vi "Publish Sample.vi"(8 "error in (no error)":errorcluster, 9 "Sample":refnum<class "Sample.lvclass">, 10 "Indice":i32[](array[numeric]), 11 "Storage Line in":refnum<class "Storage Line.lvclass">) -> (0 "error out":errorcluster, 3 "Storage Line out":refnum<class "Storage Line.lvclass">)   [LabVIEW 2015, in "cRIO-Carbondioxide.lvlib" / "CO2-Actor.lvlib" / "Storage Line.lvclass"]
uses:
  Storage Line.lvclass
  subs/Sample/Sample.lvclass
  Storage Line.lvclass/Storage Line.ctl
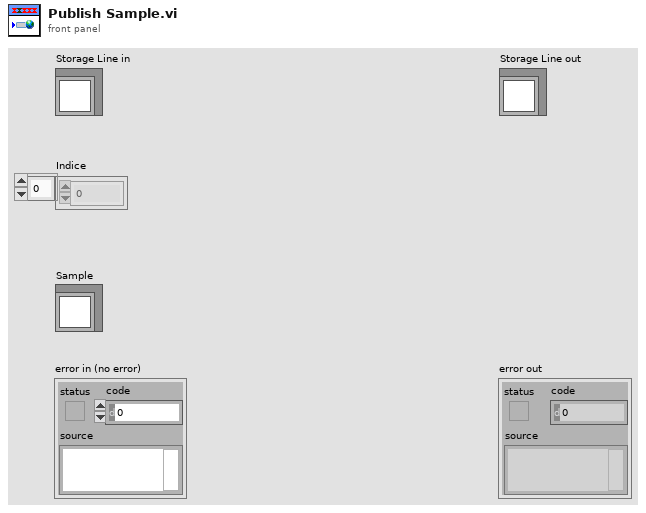
[diagram p1: front panel]
types:
  T1 = typedef "Sample Container.ctl" = cluster{"Sample In":refnum<k21>, "Sample Name":refnum<k21>, "Ti Cathode":refnum<k21>, "SampleQ":refnum<queue>}
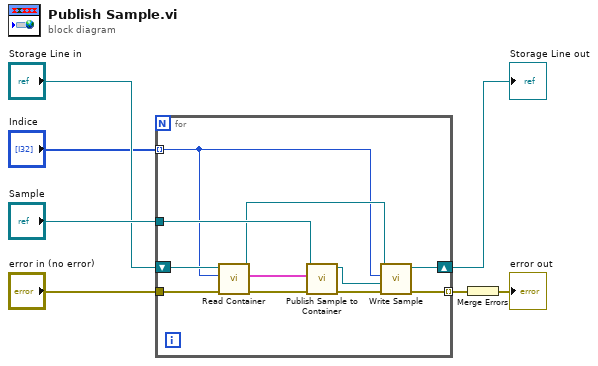
[diagram p0: block diagram]
diagram:
  n1 = for {
    tunnel: "Sample" -> [w18]
    shift-right: [w11] -> w4
    shift-left: "Storage Line in" -> [w12]
    tunnel: "Indice" -> [w9] mode=indexing
    tunnel: "error in (no error)" -> [w17]
    tunnel: [w14] -> w5 mode=indexing
    n2 = call "Read Container.vi"("error in (no error)"=w17, "index"=w9, "Storage Line in"=w12) -> ("error out"=w16:errorcluster, "Containers"=w8:T1[], "Storage Line out"=w10:refnum<class "Storage Line.lvclass">)  [unwired: 5 in, 1 out]
    n3 = call "Publish Sample to Container.vi"("error in (no error)"=w16, "Containers"=w8, "Sample in"=w18) -> ("error out"=w15:errorcluster, "Sample out"=w13:refnum<class "Sample.lvclass">)  [unwired: 7 in]
    n4 = call "Write Sample.vi"("error in (no error)"=w15, "Sample"=w13, "index"=w9, "Storage Line in"=w10) -> ("error out"=w14:errorcluster, "Storage Line out"=w11:refnum<class "Storage Line.lvclass">)  [unwired: 6 in]
  }
  "Storage Line out" <- w4
  n5 = Merge Errors(w5) -> (→"error out":errorcluster)
